vi "StringifiedData.vi"(8 "error in (no error)":errorcluster, 11 "2dStringArrayMsg in":refnum<class "2dStringArrayMsg.lvclass">) -> (0 "error out":errorcluster, 2 "Stringified Data":string, 3 "2dStringArrayMsg out":refnum<class "2dStringArrayMsg.lvclass">)   [LabVIEW 2018, in "LapDog.Messaging.v3.NativeArrays.lvlib" / "2dStringArrayMsg.lvclass"]
doc: "This VI is used for the message probe. Child classes may override it and provide the message data in string format or a short string describing the data the message contains. This string will be displayed in the probe window."
uses:
  2dStringArrayMsg.lvclass
  2dStringArrayMsg.lvclass/2dStringArrayMsg.ctl
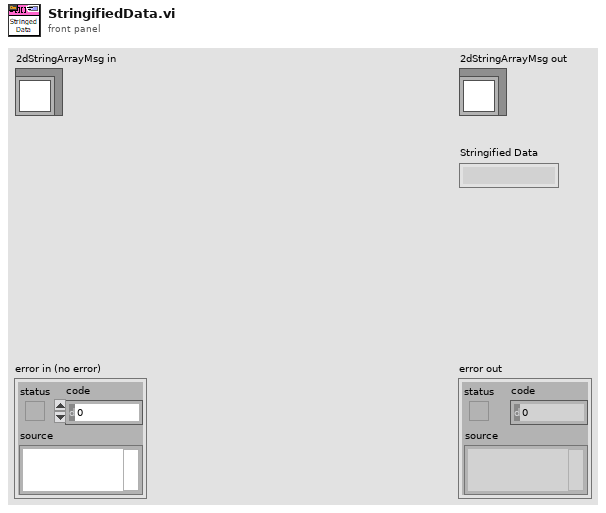
[diagram p1: front panel]
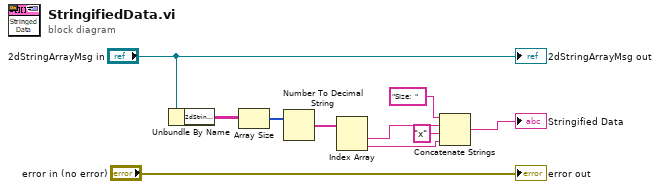
[diagram p0: block diagram]
diagram:
  n1 = Unbundle By Name("2dStringArrayMsg in") -> ("2dString[]"=w9:string[][])
  n2 = Array Size(array=w9) -> (size(s)=w8:i32[])
  n3 = Number To Decimal String(number=w8) -> (decimal integer string=w6:string[])  [unwired: 1 in]
  n4 = Index Array(array=w6) -> (element #1=w3:string, element #2=w2:string)  [unwired: 2 in]
  n5 = Concatenate Strings("Size:  " ("string"), w3, "x" ("string"), w2) -> (→"Stringified Data":string)
  "error out" <- "error in (no error)"
  "2dStringArrayMsg out" <- "2dStringArrayMsg in"
